vi "SSULE by Kamil Trajda.vi"() -> ()   [LabVIEW 2020]
uses:
  <vilib>/Utility/miscctls.llb/LVBoundsTypeDef.ctl
  <vilib>/Utility/inputDevices.llb/keyboardAcquire.vi
  <vilib>/Utility/inputDevices.llb/joystickAcquire.vi
  <vilib>/Utility/inputDevices.llb/closeJoystick.vi
  <vilib>/Utility/inputDevices.llb/closeKeyboard.vi
panel:
  out "?":bool
  in  "Przechodzenie przez ściany":bool
  in  "Rodzaj pada":string(combo)
  out "SCORE":i32
  in  "Prędkość węża":u32(slide)=150 min=150 max=200 step=1 scale=200.0..150.0
  in  "?":bool
  in  "Przechodzenie przez ściany":bool
  out "SUPER SNAKE ULTIMATE LABVIEW EDITION":picture
  # "SUPER SNAKE ULTIMATE LABVIEW EDITION !!!!"
  # "EXIT"
  # "OPCJE"
  # "Ściana"
  # "KONTROLA PADA"
  # "Używać pada?"
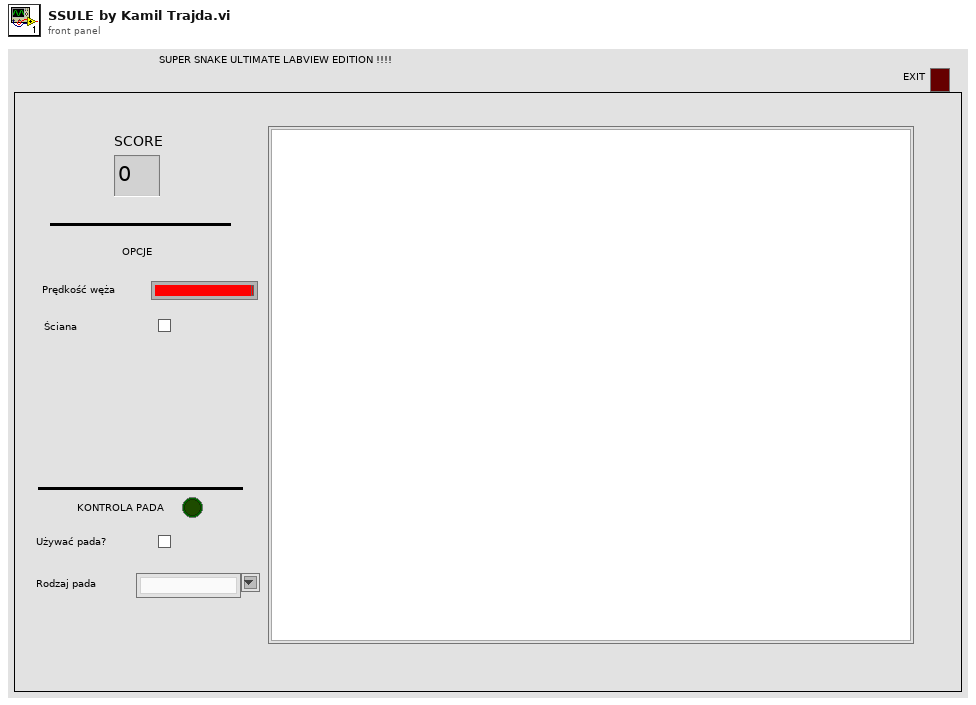
[diagram p1: front panel]
types:
  T1 = typedef "LVBoundsTypeDef.ctl" = cluster{"Width":u32, "Height":u32}
  T2 = cluster{"axes total":u32, "buttons total":u32, "pov total":u32, "device name":string}[]
  T3 = enum16{"0", "1", "2", "3", "4", "5", "6", "7", "8", "9", "A", "B", "C", "D", "E", "F", "G", "H", "I", "J", "K", "L", "M", "N", "O", "P", "Q", "R", "S", "T", "U", "V", "W", "X", "Y", "Z", "F1", "F2", "F3", "F4", "F5", "F6", "F7", "F8", "F9", "F10", "F11", "F12", "F13", "F14", "F15", "ADD", "BACK", "BACKSLASH", "CAPITAL", "COMMA", "DECIMAL", "DELETE", "DIVIDE", "DOWN", "END", "EQUALS", "ESCAPE", "GRAVE (`)", "HOME", "INSERT", "LBRACKET", "LCONTROL", "LEFT", "L ALT", "LSHIFT", "LWIN", "MINUS", "MULTIPLY", "NEXT", "NUMLOCK", "NUMPAD_0", "NUMPAD_1", "NUMPAD_2", "NUMPAD_3", "NUMPAD_4", "NUMPAD_5", "NUMPAD_6", "NUMPAD_7", "NUMPAD_8", "NUMPAD_9", "PAUSE", "PERIOD", "PRIOR (PG UP)", "RBRACKET", "RCONTROL", "RETURN", "RIGHT", "R ALT", "RSHIFT", "RWIN", "SCROLL", "SEMICOLON", "SLASH", "SPACE", "SUBTRACT", "TAB", "UP", "ENTER (num pad)", "' (quote)"}[]
  T4 = cluster{"keys pressed[0]":enum16{"0", "1", "2", "3", "4", "5", "6", "7", "8", "9", "A", "B", "C", "D", "E", "F", "G", "H", "I", "J", "K", "L", "M", "N", "O", "P", "Q", "R", "S", "T", "U", "V", "W", "X", "Y", "Z", "F1", "F2", "F3", "F4", "F5", "F6", "F7", "F8", "F9", "F10", "F11", "F12", "F13", "F14", "F15", "ADD", "BACK", "BACKSLASH", "CAPITAL", "COMMA", "DECIMAL", "DELETE", "DIVIDE", "DOWN", "END", "EQUALS", "ESCAPE", "GRAVE (`)", "HOME", "INSERT", "LBRACKET", "LCONTROL", "LEFT", "L ALT", "LSHIFT", "LWIN", "MINUS", "MULTIPLY", "NEXT", "NUMLOCK", "NUMPAD_0", "NUMPAD_1", "NUMPAD_2", "NUMPAD_3", "NUMPAD_4", "NUMPAD_5", "NUMPAD_6", "NUMPAD_7", "NUMPAD_8", "NUMPAD_9", "PAUSE", "PERIOD", "PRIOR (PG UP)", "RBRACKET", "RCONTROL", "RETURN", "RIGHT", "R ALT", "RSHIFT", "RWIN", "SCROLL", "SEMICOLON", "SLASH", "SPACE", "SUBTRACT", "TAB", "UP", "ENTER (num pad)", "' (quote)"}, "keys pressed[1]":enum16{"0", "1", "2", "3", "4", "5", "6", "7", "8", "9", "A", "B", "C", "D", "E", "F", "G", "H", "I", "J", "K", "L", "M", "N", "O", "P", "Q", "R", "S", "T", "U", "V", "W", "X", "Y", "Z", "F1", "F2", "F3", "F4", "F5", "F6", "F7", "F8", "F9", "F10", "F11", "F12", "F13", "F14", "F15", "ADD", "BACK", "BACKSLASH", "CAPITAL", "COMMA", "DECIMAL", "DELETE", "DIVIDE", "DOWN", "END", "EQUALS", "ESCAPE", "GRAVE (`)", "HOME", "INSERT", "LBRACKET", "LCONTROL", "LEFT", "L ALT", "LSHIFT", "LWIN", "MINUS", "MULTIPLY", "NEXT", "NUMLOCK", "NUMPAD_0", "NUMPAD_1", "NUMPAD_2", "NUMPAD_3", "NUMPAD_4", "NUMPAD_5", "NUMPAD_6", "NUMPAD_7", "NUMPAD_8", "NUMPAD_9", "PAUSE", "PERIOD", "PRIOR (PG UP)", "RBRACKET", "RCONTROL", "RETURN", "RIGHT", "R ALT", "RSHIFT", "RWIN", "SCROLL", "SEMICOLON", "SLASH", "SPACE", "SUBTRACT", "TAB", "UP", "ENTER (num pad)", "' (quote)"}, "keys pressed[2]":enum16{"0", "1", "2", "3", "4", "5", "6", "7", "8", "9", "A", "B", "C", "D", "E", "F", "G", "H", "I", "J", "K", "L", "M", "N", "O", "P", "Q", "R", "S", "T", "U", "V", "W", "X", "Y", "Z", "F1", "F2", "F3", "F4", "F5", "F6", "F7", "F8", "F9", "F10", "F11", "F12", "F13", "F14", "F15", "ADD", "BACK", "BACKSLASH", "CAPITAL", "COMMA", "DECIMAL", "DELETE", "DIVIDE", "DOWN", "END", "EQUALS", "ESCAPE", "GRAVE (`)", "HOME", "INSERT", "LBRACKET", "LCONTROL", "LEFT", "L ALT", "LSHIFT", "LWIN", "MINUS", "MULTIPLY", "NEXT", "NUMLOCK", "NUMPAD_0", "NUMPAD_1", "NUMPAD_2", "NUMPAD_3", "NUMPAD_4", "NUMPAD_5", "NUMPAD_6", "NUMPAD_7", "NUMPAD_8", "NUMPAD_9", "PAUSE", "PERIOD", "PRIOR (PG UP)", "RBRACKET", "RCONTROL", "RETURN", "RIGHT", "R ALT", "RSHIFT", "RWIN", "SCROLL", "SEMICOLON", "SLASH", "SPACE", "SUBTRACT", "TAB", "UP", "ENTER (num pad)", "' (quote)"}, "keys pressed[3]":enum16{"0", "1", "2", "3", "4", "5", "6", "7", "8", "9", "A", "B", "C", "D", "E", "F", "G", "H", "I", "J", "K", "L", "M", "N", "O", "P", "Q", "R", "S", "T", "U", "V", "W", "X", "Y", "Z", "F1", "F2", "F3", "F4", "F5", "F6", "F7", "F8", "F9", "F10", "F11", "F12", "F13", "F14", "F15", "ADD", "BACK", "BACKSLASH", "CAPITAL", "COMMA", "DECIMAL", "DELETE", "DIVIDE", "DOWN", "END", "EQUALS", "ESCAPE", "GRAVE (`)", "HOME", "INSERT", "LBRACKET", "LCONTROL", "LEFT", "L ALT", "LSHIFT", "LWIN", "MINUS", "MULTIPLY", "NEXT", "NUMLOCK", "NUMPAD_0", "NUMPAD_1", "NUMPAD_2", "NUMPAD_3", "NUMPAD_4", "NUMPAD_5", "NUMPAD_6", "NUMPAD_7", "NUMPAD_8", "NUMPAD_9", "PAUSE", "PERIOD", "PRIOR (PG UP)", "RBRACKET", "RCONTROL", "RETURN", "RIGHT", "R ALT", "RSHIFT", "RWIN", "SCROLL", "SEMICOLON", "SLASH", "SPACE", "SUBTRACT", "TAB", "UP", "ENTER (num pad)", "' (quote)"}, "keys pressed[4]":enum16{"0", "1", "2", "3", "4", "5", "6", "7", "8", "9", "A", "B", "C", "D", "E", "F", "G", "H", "I", "J", "K", "L", "M", "N", "O", "P", "Q", "R", "S", "T", "U", "V", "W", "X", "Y", "Z", "F1", "F2", "F3", "F4", "F5", "F6", "F7", "F8", "F9", "F10", "F11", "F12", "F13", "F14", "F15", "ADD", "BACK", "BACKSLASH", "CAPITAL", "COMMA", "DECIMAL", "DELETE", "DIVIDE", "DOWN", "END", "EQUALS", "ESCAPE", "GRAVE (`)", "HOME", "INSERT", "LBRACKET", "LCONTROL", "LEFT", "L ALT", "LSHIFT", "LWIN", "MINUS", "MULTIPLY", "NEXT", "NUMLOCK", "NUMPAD_0", "NUMPAD_1", "NUMPAD_2", "NUMPAD_3", "NUMPAD_4", "NUMPAD_5", "NUMPAD_6", "NUMPAD_7", "NUMPAD_8", "NUMPAD_9", "PAUSE", "PERIOD", "PRIOR (PG UP)", "RBRACKET", "RCONTROL", "RETURN", "RIGHT", "R ALT", "RSHIFT", "RWIN", "SCROLL", "SEMICOLON", "SLASH", "SPACE", "SUBTRACT", "TAB", "UP", "ENTER (num pad)", "' (quote)"}, "keys pressed[5]":enum16{"0", "1", "2", "3", "4", "5", "6", "7", "8", "9", "A", "B", "C", "D", "E", "F", "G", "H", "I", "J", "K", "L", "M", "N", "O", "P", "Q", "R", "S", "T", "U", "V", "W", "X", "Y", "Z", "F1", "F2", "F3", "F4", "F5", "F6", "F7", "F8", "F9", "F10", "F11", "F12", "F13", "F14", "F15", "ADD", "BACK", "BACKSLASH", "CAPITAL", "COMMA", "DECIMAL", "DELETE", "DIVIDE", "DOWN", "END", "EQUALS", "ESCAPE", "GRAVE (`)", "HOME", "INSERT", "LBRACKET", "LCONTROL", "LEFT", "L ALT", "LSHIFT", "LWIN", "MINUS", "MULTIPLY", "NEXT", "NUMLOCK", "NUMPAD_0", "NUMPAD_1", "NUMPAD_2", "NUMPAD_3", "NUMPAD_4", "NUMPAD_5", "NUMPAD_6", "NUMPAD_7", "NUMPAD_8", "NUMPAD_9", "PAUSE", "PERIOD", "PRIOR (PG UP)", "RBRACKET", "RCONTROL", "RETURN", "RIGHT", "R ALT", "RSHIFT", "RWIN", "SCROLL", "SEMICOLON", "SLASH", "SPACE", "SUBTRACT", "TAB", "UP", "ENTER (num pad)", "' (quote)"}, "keys pressed[6]":enum16{"0", "1", "2", "3", "4", "5", "6", "7", "8", "9", "A", "B", "C", "D", "E", "F", "G", "H", "I", "J", "K", "L", "M", "N", "O", "P", "Q", "R", "S", "T", "U", "V", "W", "X", "Y", "Z", "F1", "F2", "F3", "F4", "F5", "F6", "F7", "F8", "F9", "F10", "F11", "F12", "F13", "F14", "F15", "ADD", "BACK", "BACKSLASH", "CAPITAL", "COMMA", "DECIMAL", "DELETE", "DIVIDE", "DOWN", "END", "EQUALS", "ESCAPE", "GRAVE (`)", "HOME", "INSERT", "LBRACKET", "LCONTROL", "LEFT", "L ALT", "LSHIFT", "LWIN", "MINUS", "MULTIPLY", "NEXT", "NUMLOCK", "NUMPAD_0", "NUMPAD_1", "NUMPAD_2", "NUMPAD_3", "NUMPAD_4", "NUMPAD_5", "NUMPAD_6", "NUMPAD_7", "NUMPAD_8", "NUMPAD_9", "PAUSE", "PERIOD", "PRIOR (PG UP)", "RBRACKET", "RCONTROL", "RETURN", "RIGHT", "R ALT", "RSHIFT", "RWIN", "SCROLL", "SEMICOLON", "SLASH", "SPACE", "SUBTRACT", "TAB", "UP", "ENTER (num pad)", "' (quote)"}, "keys pressed[7]":enum16{"0", "1", "2", "3", "4", "5", "6", "7", "8", "9", "A", "B", "C", "D", "E", "F", "G", "H", "I", "J", "K", "L", "M", "N", "O", "P", "Q", "R", "S", "T", "U", "V", "W", "X", "Y", "Z", "F1", "F2", "F3", "F4", "F5", "F6", "F7", "F8", "F9", "F10", "F11", "F12", "F13", "F14", "F15", "ADD", "BACK", "BACKSLASH", "CAPITAL", "COMMA", "DECIMAL", "DELETE", "DIVIDE", "DOWN", "END", "EQUALS", "ESCAPE", "GRAVE (`)", "HOME", "INSERT", "LBRACKET", "LCONTROL", "LEFT", "L ALT", "LSHIFT", "LWIN", "MINUS", "MULTIPLY", "NEXT", "NUMLOCK", "NUMPAD_0", "NUMPAD_1", "NUMPAD_2", "NUMPAD_3", "NUMPAD_4", "NUMPAD_5", "NUMPAD_6", "NUMPAD_7", "NUMPAD_8", "NUMPAD_9", "PAUSE", "PERIOD", "PRIOR (PG UP)", "RBRACKET", "RCONTROL", "RETURN", "RIGHT", "R ALT", "RSHIFT", "RWIN", "SCROLL", "SEMICOLON", "SLASH", "SPACE", "SUBTRACT", "TAB", "UP", "ENTER (num pad)", "' (quote)"}, "keys pressed[8]":enum16{"0", "1", "2", "3", "4", "5", "6", "7", "8", "9", "A", "B", "C", "D", "E", "F", "G", "H", "I", "J", "K", "L", "M", "N", "O", "P", "Q", "R", "S", "T", "U", "V", "W", "X", "Y", "Z", "F1", "F2", "F3", "F4", "F5", "F6", "F7", "F8", "F9", "F10", "F11", "F12", "F13", "F14", "F15", "ADD", "BACK", "BACKSLASH", "CAPITAL", "COMMA", "DECIMAL", "DELETE", "DIVIDE", "DOWN", "END", "EQUALS", "ESCAPE", "GRAVE (`)", "HOME", "INSERT", "LBRACKET", "LCONTROL", "LEFT", "L ALT", "LSHIFT", "LWIN", "MINUS", "MULTIPLY", "NEXT", "NUMLOCK", "NUMPAD_0", "NUMPAD_1", "NUMPAD_2", "NUMPAD_3", "NUMPAD_4", "NUMPAD_5", "NUMPAD_6", "NUMPAD_7", "NUMPAD_8", "NUMPAD_9", "PAUSE", "PERIOD", "PRIOR (PG UP)", "RBRACKET", "RCONTROL", "RETURN", "RIGHT", "R ALT", "RSHIFT", "RWIN", "SCROLL", "SEMICOLON", "SLASH", "SPACE", "SUBTRACT", "TAB", "UP", "ENTER (num pad)", "' (quote)"}}
  T5 = enum16{"0", "1", "2", "3", "4", "5", "6", "7", "8", "9", "A", "B", "C", "D", "E", "F", "G", "H", "I", "J", "K", "L", "M", "N", "O", "P", "Q", "R", "S", "T", "U", "V", "W", "X", "Y", "Z", "F1", "F2", "F3", "F4", "F5", "F6", "F7", "F8", "F9", "F10", "F11", "F12", "F13", "F14", "F15", "ADD", "BACK", "BACKSLASH", "CAPITAL", "COMMA", "DECIMAL", "DELETE", "DIVIDE", "DOWN", "END", "EQUALS", "ESCAPE", "GRAVE (`)", "HOME", "INSERT", "LBRACKET", "LCONTROL", "LEFT", "L ALT", "LSHIFT", "LWIN", "MINUS", "MULTIPLY", "NEXT", "NUMLOCK", "NUMPAD_0", "NUMPAD_1", "NUMPAD_2", "NUMPAD_3", "NUMPAD_4", "NUMPAD_5", "NUMPAD_6", "NUMPAD_7", "NUMPAD_8", "NUMPAD_9", "PAUSE", "PERIOD", "PRIOR (PG UP)", "RBRACKET", "RCONTROL", "RETURN", "RIGHT", "R ALT", "RSHIFT", "RWIN", "SCROLL", "SEMICOLON", "SLASH", "SPACE", "SUBTRACT", "TAB", "UP", "ENTER (num pad)", "' (quote)"}
  T6 = cluster{"X axis":i32, "Y axis":i32, "Z axis":i32, "X axis rotation":i32, "Y axis rotation":i32, "Z axis rotation":i32, "U axis":i32, "V axis":i32}
  T7 = typedef "imagedata.ctl" = cluster{"image type":i32, "image depth":i32, "image":u8[], "mask":u8[], "colors":u32[], "Rectangle":cluster{"left":i16, "top":i16, "right":i16, "bottom":i16}}
  T8 = cluster{"image type":i32, "image depth":i32, "image":u8[], "mask":u8[], "colors":u32[], "Cluster":cluster{dbl, dbl, dbl, dbl}}
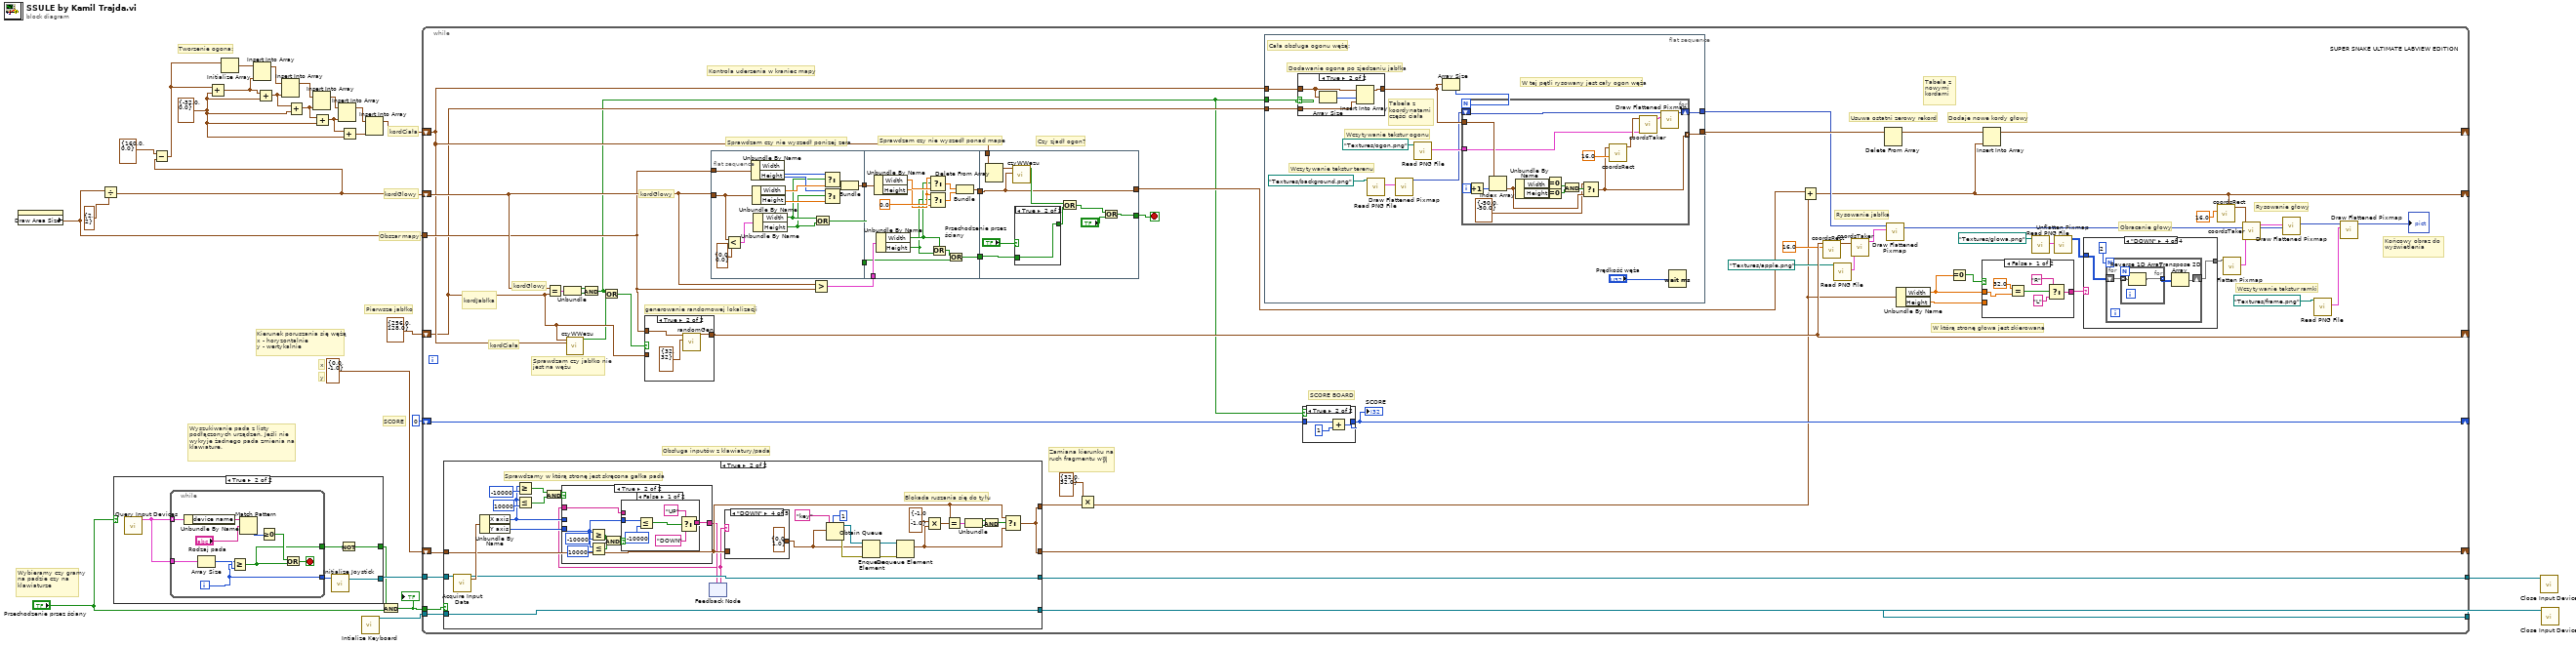
[diagram p0: block diagram]
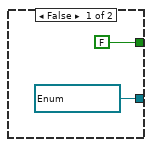
[diagram p2: hidden frame]
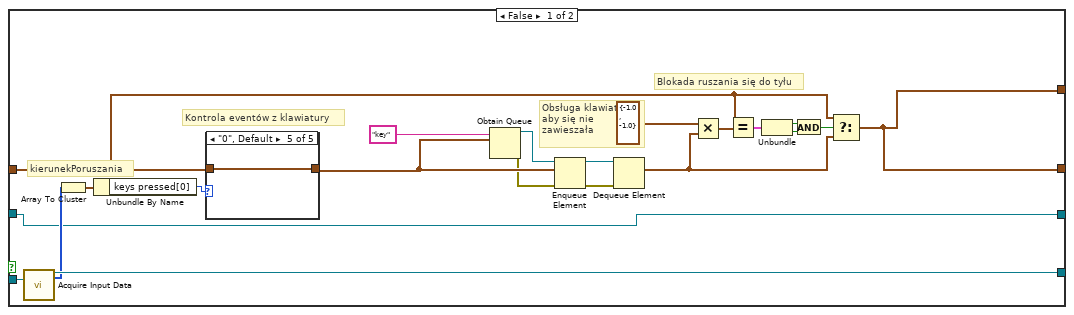
[diagram p3: hidden frame]
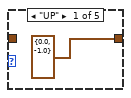
[diagram p4: hidden frame]
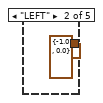
[diagram p5: hidden frame]
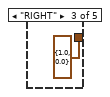
[diagram p6: hidden frame]
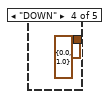
[diagram p7: hidden frame]
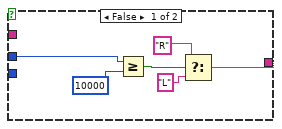
[diagram p8: hidden frame]
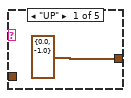
[diagram p10: hidden frame]
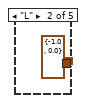
[diagram p11: hidden frame]
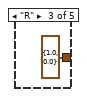
[diagram p12: hidden frame]
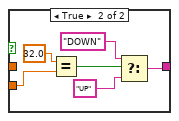
[diagram p15: hidden frame]
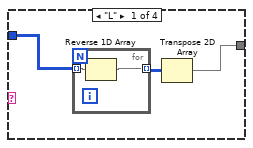
[diagram p16: hidden frame]
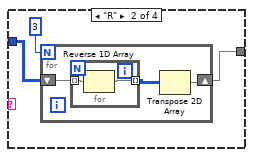
[diagram p17: hidden frame]
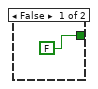
[diagram p20: hidden frame]
diagram:
  w16 = cluster{"Width":dbl, "Height":dbl} {"Width"=-32.0, "Height"=0.0} ("y")
  # "SCORE"
  # "Wyszukiwanie pada z listy podłączonych urządzeń. Jeśli nie wykryje żadnego pada zmienia na klawiature."
  # "Wybieramy czy gramy na padzie czy na klawiaturze"
  # "kordCiała"
  # "Obszar mapy"
  # "kordGlowy"
  # "Pierwsze jabłko"
  # "y"
  # "x"
  # "Kierunek poruszania się wężą\nx - horyzontalnie\ny - wertykalnie"
  # "Tworzenie ogona:"
  n1 = property class="Pict"() -> ("Draw Area Size"=w26:T1)  [unwired: 2 in, 2 out]
  n2 = Divide(x=w26, y=T1 {"Width"=2, "Height"=2}) -> (x/y=w10:cluster{"Width":dbl, "Height":dbl})
  n3 = case shown="True" "Przechodzenie przez ściany" {
    tunnel: [w29 w34] -> w6
    tunnel: [FALSE w31] -> w3
    frame False {
      w29 = refnum<k1> refnum items=["JOYSTICK"] ("device ID")
    }
    frame True {
      n4 = call <vilib>:"Query Input Devices.vi"() -> ("joystick info"=w33:T2)  [unwired: 8 in, 3 out]
      n5 = while {
        tunnel: w33 -> [w42] mode=indexing
        tunnel: w33 -> [w44]
        tunnel: [w38] -> w30
        tunnel: [w36] -> w32
        i -> [w36]
        stop <- w40 stop-if-true
        n6 = Unbundle By Name(w42) -> ("device name"=w35:string)
        n7 = Array Size(array=w44) -> (size(s)=w37:i32)
        n8 = Greater Or Equal?(x=w36, y=w37) -> (x >= y?=w38:bool)
        n9 = Match Pattern(string=w35, regular expression="Rodzaj pada") -> (offset past match=w41:i32)  [unwired: 1 in, 3 out]
        n10 = Greater Or Equal To 0?(x=w41) -> (x >= 0?=w39:bool)
        n11 = Or(x=w39, y=w38) -> (x .or. y?=w40:bool)
      }
      n12 = call <vilib>:"Initialize Joystick.vi"("device index"=w32) -> ("device ID"=w34:refnum<k1>)  [unwired: 9 in, 1 out]
      n13 = Not(x=w30) -> (.not. x?=w31:bool)
    }
  }
  n14 = Subtract(x=cluster{"Width":dbl, "Height":dbl} {"Width"=160.0, "Height"=0.0} ("y"), y=w10) -> (x-y=w8:cluster{"Width":dbl, "Height":dbl})
  n15 = Add(x=w8, y=w16) -> (x+y=w21:cluster{"Width":dbl, "Height":dbl})
  n16 = Initialize Array(w8) -> (w23:cluster{"Width":dbl, "Height":dbl}[])  [unwired: 1 in]
  n17 = Insert Into Array(array=w23, new element=w21) -> (w22:cluster{"Width":dbl, "Height":dbl}[])  [unwired: 1 in]
  n18 = Add(x=w21, y=w16) -> (x+y=w19:cluster{"Width":dbl, "Height":dbl})
  n19 = Insert Into Array(array=w22, new element=w19) -> (w15:cluster{"Width":dbl, "Height":dbl}[])  [unwired: 1 in]
  n20 = Add(x=w19, y=w16) -> (x+y=w18:cluster{"Width":dbl, "Height":dbl})
  n21 = Insert Into Array(array=w15, new element=w18) -> (w14:cluster{"Width":dbl, "Height":dbl}[])  [unwired: 1 in]
  n22 = Add(x=w18, y=w16) -> (x+y=w17:cluster{"Width":dbl, "Height":dbl})
  n23 = Insert Into Array(array=w14, new element=w17) -> (w13:cluster{"Width":dbl, "Height":dbl}[])  [unwired: 1 in]
  n24 = Add(x=w17, y=w16) -> (x+y=w20:cluster{"Width":dbl, "Height":dbl})
  n25 = call <vilib>:"Intialize Keyboard.vi"() -> ("device ID"=w4:refnum<k1>)  [unwired: 10 in, 1 out]
  n26 = Insert Into Array(array=w13, new element=w20) -> (w12:cluster{"Width":dbl, "Height":dbl}[])  [unwired: 1 in]
  n27 = And(x=w3, y="Przechodzenie przez ściany") -> (x .and. y?=w1:bool)
  "?" <- w1
  n28 = while {
    shift-right: [w60] -> _
    shift-left: w10 -> [w95]
    tunnel: w26 -> [w94]
    tunnel: w4 -> [w101]
    tunnel: [w100] -> w25
    shift-right: [w96] -> _
    shift-left: cluster{"Width":dbl, "Height":dbl} {"Width"=0.0, "Height"=-1.0} ("y") -> [w97]
    shift-right: [w99] -> _
    shift-left: w12 -> [w93]
    shift-right: [w67] -> _
    shift-left: cluster{dbl, dbl} {256.0, 128.0} -> [w92]
    shift-right: [w55] -> _
    shift-left: 0 -> [w56]
    tunnel: w6 -> [w50]
    tunnel: w1 -> [w49]
    tunnel: [w48] -> w5
    stop <- w79 stop-if-true
    # "Końcowy obraz do wyświetlenia"
    # "Zamiana kierunku na ruch fragmentu w꿹"
    # "Obsługa inputów z klawiatury/pada"
    # "Wczytywanie tekstur ramki"
    # "SCORE BOARD"
    # "Obracanie głowy"
    # "W którą stronę głowa jest skierowana"
    # "Rysowanie jabłka"
    # "Czy zjadł ogon?"
    # "Sprawdzam czy nie wyszedł ponizej zera"
    # "Sprawdzam czy nie wyszedł ponad mape"
    # "kordCiała"
    # "kordJabłka"
    # "kordGlowy"
    # "kordGlowy"
    # "Sprawdzam czy jabłko nie jest na wężu"
    # "generowanie randomowej lokalizacji"
    # "Kontrola uderzenia w kraniec mapy"
    # "Dodaje nowe kordy głowy"
    # "Usuwa ostatni zerowy rekord"
    # "Tabela z nowymi kordami"
    # "Rysowanie głowy"
    n29 = case shown="True" w49 {
      tunnel: w101 -> [w122 w154]
      tunnel: [w121 w154] -> w100
      tunnel: w97 -> [w105 w138]
      tunnel: [w102 w139] -> w96
      tunnel: [w102 w139] -> w46
      tunnel: w50 -> [w103 w156]
      tunnel: [w103 w153] -> w48
      frame False {
        # "kierunekPoruszania"
        # "Blokada ruszania się do tyłu"
        # "Obsługa klawiatury, aby się nie zawieszała"
        # "Kontrola eventów z klawiatury"
        n30 = call-poly <vilib>:"Acquire Input Data.vi"("device ID"=w122) -> ("device ID"=w121:refnum<k1>, "keys pressed"=w120:T3)  [unwired: 16 in, 1 out]
        n31 = Array To Cluster(array=w120) -> (cluster=w119:T4)
        n32 = Unbundle By Name(w119) -> ("keys pressed[0]"=w118:T5)
        n33 = case shown="\"0\", Default" w118 {
          tunnel: [cluster{"Width":dbl, "Height":dbl} {"Width"=0.0, "Height"=-1.0} ("y") cluster{"Width":dbl, "Height":dbl} {"Width"=-1.0, "Height"=0.0} ("y") cluster{"Width":dbl, "Height":dbl} {"Width"=1.0, "Height"=0.0} ("y") cluster{"Width":dbl, "Height":dbl} {"Width"=0.0, "Height"=1.0} ("y") w127] -> w117
          tunnel: w105 -> [_ _ _ _ w127]
          frame "UP" {
          }
          frame "LEFT" {
          }
          frame "RIGHT" {
          }
          frame "DOWN" {
          }
          frame "0", Default {
          }
        }
        n34 = Obtain Queue(name (unnamed)="key", element data type=w117) -> (queue out=w116:refnum<queue>, error out=w114:errorcluster)  [unwired: 3 in, 1 out]
        n35 = Enqueue Element(queue=w116, element=w117, error in (no error)=w114) -> (queue out=w115:refnum<queue>, error out=w113:errorcluster)  [unwired: 1 in, 1 out]
        n36 = Dequeue Element(queue=w115, error in (no error)=w113) -> (element=w104:cluster{"Width":dbl, "Height":dbl})  [unwired: 1 in, 3 out]
        n37 = Multiply(x=cluster{"Width":dbl, "Height":dbl} {"Width"=-1.0, "Height"=-1.0}, y=w104) -> (x*y=w111:cluster{"Width":dbl, "Height":dbl})
        n38 = Equal?(x=w105, y=w111) -> (x = y?=w107:cluster{"Width":bool, "Height":bool})
        n39 = Unbundle(w107) -> ("Width"=w109:bool, "Height"=w108:bool)
        n40 = And(x=w109, y=w108) -> (x .and. y?=w106:bool)
        n41 = Select(t=w105, s=w106, f=w104) -> (s? t:f=w102:cluster{"Width":dbl, "Height":dbl})
      }
      frame True {
        # "Sprawdzamy w którą stronę jest skręcona gałka pada"
        # "Blokada ruszania się do tyłu"
        n42 = call-poly <vilib>:"Acquire Input Data.vi"("device ID"=w156) -> ("device ID"=w153:refnum<k1>, "axis info"=w155:T6)  [unwired: 14 in, 3 out]
        n43 = Unbundle By Name(w155) -> ("X axis"=w147:i32, "Y axis"=w146:i32)
        n44 = Greater Or Equal?(x=w147, y=-10000) -> (x >= y?=w152:bool)
        n45 = Less Or Equal?(x=w147, y=10000) -> (x <= y?=w151:bool)
        n46 = And(x=w152, y=w151) -> (x .and. y?=w148:bool)
        n47 = feedback #1() -> (w129:string)  [unwired: 1 in]
        n48 = case shown="True" w148 {
          tunnel: w147 -> [w157 _]
          tunnel: w146 -> [_ w165]
          tunnel: [w160 w164] -> w130
          tunnel: w129 -> [_ w163]
          frame False {
            n49 = Greater Or Equal?(x=w157, y=10000) -> (x >= y?=w158:bool)
            n50 = Select(t="R", s=w158, f="L") -> (s? t:f=w160:string)
          }
          frame True {
            n51 = Greater Or Equal?(x=w165, y=-10000) -> (x >= y?=w170:bool)
            n52 = Less Or Equal?(x=w165, y=10000) -> (x <= y?=w169:bool)
            n53 = And(x=w170, y=w169) -> (x .and. y?=w166:bool)
            n54 = case shown="False" w166 {
              tunnel: w165 -> [w172 _]
              tunnel: [w171 w177] -> w164
              tunnel: w163 -> [_ w177]
              frame False {
                n55 = Less Or Equal?(x=w172, y=-10000) -> (x <= y?=w176:bool)
                n56 = Select(t="UP", s=w176, f="DOWN") -> (s? t:f=w171:string)
              }
              frame True {
              }
            }
          }
        }
        n57 = feedback-in #1(w130) -> ()
        n58 = case shown="\"DOWN\"" w129 {
          tunnel: [cluster{"Width":dbl, "Height":dbl} {"Width"=0.0, "Height"=-1.0} ("y") cluster{"Width":dbl, "Height":dbl} {"Width"=-1.0, "Height"=0.0} ("y") cluster{"Width":dbl, "Height":dbl} {"Width"=1.0, "Height"=0.0} ("y") cluster{"Width":dbl, "Height":dbl} {"Width"=0.0, "Height"=1.0} ("y") w182] -> w132
          tunnel: w138 -> [_ _ _ _ w182]
          frame "UP" {
          }
          frame "L" {
          }
          frame "R" {
          }
          frame "DOWN" {
          }
          frame "0", Default {
          }
        }
        n59 = Obtain Queue(max queue size (-1, unlimited)=1, name (unnamed)="key", element data type=w132) -> (queue out=w137:refnum<queue>, error out=w135:errorcluster)  [unwired: 2 in, 1 out]
        n60 = Enqueue Element(queue=w137, element=w132, error in (no error)=w135) -> (queue out=w136:refnum<queue>, error out=w134:errorcluster)  [unwired: 1 in, 1 out]
        n61 = Dequeue Element(queue=w136, error in (no error)=w134) -> (element=w131:cluster{"Width":dbl, "Height":dbl})  [unwired: 1 in, 3 out]
        n62 = Multiply(x=cluster{"Width":dbl, "Height":dbl} {"Width"=-1.0, "Height"=-1.0}, y=w131) -> (x*y=w145:cluster{"Width":dbl, "Height":dbl})
        n63 = Equal?(x=w138, y=w145) -> (x = y?=w141:cluster{"Width":bool, "Height":bool})
        n64 = Unbundle(w141) -> ("Width"=w143:bool, "Height"=w142:bool)
        n65 = And(x=w143, y=w142) -> (x .and. y?=w140:bool)
        n66 = Select(t=w138, s=w140, f=w131) -> (s? t:f=w139:cluster{"Width":dbl, "Height":dbl})
      }
    }
    n67 = Equal?(x=w95, y=w92) -> (x = y?=w85:cluster{bool, bool})
    n68 = Unbundle(w85) -> (w84:bool, w83:bool)
    n69 = call "czyWWezu.vi"("kordyPunktu"=w92, "kordyCiala"=w93) -> ("czyNaszedl?"=w81:bool)  [unwired: 9 in]
    n70 = And(x=w84, y=w83) -> (x .and. y?=w57:bool)
    n71 = Or(x=w57, y=w81) -> (x .or. y?=w82:bool)
    n72 = case shown="True" w82 {
      tunnel: w94 -> [_ w298]
      tunnel: [w295 w297] -> w67
      tunnel: w92 -> [w295 _]
      frame False {
      }
      frame True {
        n73 = call "randomGen.vi"("dzielnikMapy"=T1 {"Width"=32, "Height"=32} ("y"), "Wielkosc mapy"=w298) -> ("wygenerowane współrzędne"=w297:cluster{u64, u64})  [unwired: 9 in]
      }
    }
    n74 = flat-sequence {
      tunnel: w94 -> [w269]
      tunnel: w95 -> [w259]
      tunnel: [w262] -> w89
      tunnel: [w256] -> w88
      tunnel: w89 -> [w278]
      tunnel: w80 -> [w282]
      tunnel: [w279] -> w87
      tunnel: w88 -> [w271]
      tunnel: [w270] -> w86
      tunnel: [w289] -> w90
      tunnel: w87 -> [w289]
      tunnel: w93 -> [w291]
      tunnel: w86 -> [w287]
      tunnel: [w283] -> w79
      frame #0 {
        n75 = Less?(x=w259, y=cluster{"Width":dbl, "Height":dbl} {"Width"=0.0, "Height"=0.0}) -> (x < y?=w261:cluster{"Width":bool, "Height":bool})
        n76 = Unbundle By Name(w269) -> ("Width"=w268:u32, "Height"=w265:u32)
        n77 = Unbundle By Name(w259) -> ("Width"=w267:dbl, "Height"=w266:dbl)
        n78 = Unbundle By Name(w261) -> ("Width"=w258:bool, "Height"=w257:bool)
        n79 = Or(x=w258, y=w257) -> (x .or. y?=w256:bool)
        n80 = Select(t=w268, s=w258, f=w267) -> (s? t:f=w264:dbl)
        n81 = Select(t=w265, s=w257, f=w266) -> (s? t:f=w263:dbl)
        n82 = Bundle("Width"=w264, "Height"=w263) -> (w262:cluster{"Width":dbl, "Height":dbl})  [unwired: 1 in]
      }
      frame #1 {
        w276 = 0.0 ("f")
        n83 = Unbundle By Name(w278) -> ("Width"=w277:dbl, "Height"=w275:dbl)
        n84 = Unbundle By Name(w282) -> ("Width"=w274:bool, "Height"=w273:bool)
        n85 = Select(t=w276, s=w274, f=w277) -> (s? t:f=w281:dbl)
        n86 = Select(t=w276, s=w273, f=w275) -> (s? t:f=w280:dbl)
        n87 = Or(x=w274, y=w273) -> (x .or. y?=w272:bool)
        n88 = Or(x=w272, y=w271) -> (x .or. y?=w270:bool)
        n89 = Bundle("Width"=w281, "Height"=w280) -> (w279:cluster{"Width":dbl, "Height":dbl})  [unwired: 1 in]
      }
      frame #2 {
        n90 = Delete From Array(array=w291) -> (array with subset deleted=w292:cluster{"Width":dbl, "Height":dbl}[])  [unwired: 2 in, 1 out]
        n91 = call "czyWWezu.vi"("kordyPunktu"=w289, "kordyCiala"=w292) -> ("czyNaszedl?"=w290:bool)  [unwired: 9 in]
        n92 = case shown="True" "Przechodzenie przez ściany" {
          tunnel: w287 -> [_ w294]
          tunnel: [FALSE w294] -> w286
          frame False {
          }
          frame True {
          }
        }
        n93 = Or(x=w290, y=w286) -> (x .or. y?=w284:bool)
        n94 = Or(x=w284, y="?") -> (x .or. y?=w283:bool)
      }
    }
    n95 = Greater?(x=w95, y=w94) -> (0:w80:cluster{"Width":bool, "Height":bool})
    n96 = Multiply(x=cluster{"Width":dbl, "Height":dbl} {"Width"=32.0, "Height"=32.0} ("y"), y=w46) -> (x*y=w45:cluster{"Width":dbl, "Height":dbl})
    n97 = flat-sequence {
      tunnel: w57 -> [w233]
      tunnel: w93 -> [w232]
      tunnel: w92 -> [w231]
      tunnel: [w230] -> w62
      tunnel: [w229] -> w91
      frame #0 {
        # "Wczytywanie tekstur ogonu"
        # "Wczytywanie tekstur terenu"
        # "Dodawanie ogona po zjedzeniu jabłka"
        # "Tabela z koordynatami\nczęści ciała"
        # "W tej pętli rysowany jest cały ogon węża"
        # "Cała obsługa ogonu wężą:"
        n98 = case shown="True" w233 {
          tunnel: w232 -> [w234 w236]
          tunnel: [w234 w238] -> w228
          tunnel: w231 -> [_ w235]
          frame False {
          }
          frame True {
            n99 = Array Size(array=w236) -> (size(s)=w237:i32)
            n100 = Insert Into Array(array=w236, index=w237, new element=w235) -> (w238:cluster{"Width":dbl, "Height":dbl}[])
          }
        }
        n101 = call <vilib>:"Read PNG File.vi"("path to PNG file"=path "Textures/background.png") -> ("image data"=w223:T7)  [unwired: 8 in, 2 out]
        n102 = call <vilib>:"Draw Flattened Pixmap.vi"("image data"=w223) -> ("new picture"=w221:picture)  [unwired: 8 in]
        n103 = call <vilib>:"Read PNG File.vi"("path to PNG file"=path "Textures/ogon.png") -> ("image data"=w224:T7)  [unwired: 8 in, 2 out]
        n104 = Array Size(array=w228) -> (size(s)=w227:i32)
        n105 = for {
          N: w227 -> [_]
          shift-right: [w240] -> w230
          shift-left: w221 -> [w241]
          tunnel: w228 -> [w255]
          tunnel: [w244] -> w229 mode=indexing
          tunnel: w224 -> [w239]
          i -> [w253]
          n106 = Increment(x=w253) -> (x+1=w254:i32)
          n107 = Index Array(array=w255, index=w254) -> (element=w247:cluster{"Width":dbl, "Height":dbl})
          n108 = Unbundle By Name(w247) -> ("Width"=w252:dbl, "Height"=w251:dbl)
          n109 = Equal To 0?(x=w252) -> (x = 0?=w250:bool)
          n110 = Equal To 0?(x=w251) -> (x = 0?=w249:bool)
          n111 = And(x=w250, y=w249) -> (x .and. y?=w248:bool)
          n112 = Select(t=cluster{"Width":dbl, "Height":dbl} {"Width"=-50.0, "Height"=-50.0}, s=w248, f=w247) -> (s? t:f=w244:cluster{"Width":dbl, "Height":dbl})
          n113 = call "coordsRect.vi"("Rozmiar"=16.0 ("liczba"), "coords"=w244) -> ("Cluster"=w242:cluster{dbl, dbl, dbl, dbl})  [unwired: 9 in]
          n114 = call "coordsTaker.vi"("image data"=w239, "coords"=w242) -> ("Cluster out"=w243:T8)  [unwired: 9 in]
          n115 = call <vilib>:"Draw Flattened Pixmap.vi"("image data"=w243, "picture"=w241) -> ("new picture"=w240:picture)  [unwired: 7 in]
        }
        n116 = Wait (ms)(milliseconds to wait="Prędkość węża") -> ()  [unwired: 1 out]
      }
    }
    n117 = case shown="True" w57 {
      tunnel: w56 -> [w183 w186]
      tunnel: [w183 w185] -> w55
      frame False {
      }
      frame True {
        n118 = Add(x=w186, y=1) -> (x+y=w185:i32)
      }
    }
    "SCORE" <- w55
    n119 = Add(x=w90, y=w45) -> (x+y=w60:cluster{"Width":dbl, "Height":dbl})
    n120 = call "coordsRect.vi"("Rozmiar"=16.0, "coords"=w67) -> ("Cluster"=w64:cluster{dbl, dbl, dbl, dbl})  [unwired: 9 in]
    n121 = call <vilib>:"Read PNG File.vi"("path to PNG file"=path "Textures/apple.png") -> ("image data"=w59:T7)  [unwired: 8 in, 2 out]
    n122 = call "coordsTaker.vi"("image data"=w59, "coords"=w64) -> ("Cluster out"=w61:T8)  [unwired: 9 in]
    n123 = Delete From Array(array=w91) -> (array with subset deleted=w98:cluster{"Width":dbl, "Height":dbl}[])  [unwired: 2 in, 1 out]
    n124 = call <vilib>:"Draw Flattened Pixmap.vi"("image data"=w61, "picture"=w62) -> ("new picture"=w63:picture)  [unwired: 7 in]
    n125 = Unbundle By Name(w45) -> ("Width"=w69:dbl, "Height"=w70:dbl)
    n126 = Equal To 0?(x=w69) -> (x = 0?=w71:bool)
    n127 = case shown="False" w71 {
      tunnel: w70 -> [_ w197]
      tunnel: [w189 w193] -> w68
      tunnel: w69 -> [w190 _]
      frame False {
        n128 = Equal?(x=32.0, y=w190) -> (x = y?=w192:bool)
        n129 = Select(t="R", s=w192, f="L") -> (s? t:f=w189:string)
      }
      frame True {
        n130 = Equal?(x=32.0, y=w197) -> (x = y?=w198:bool)
        n131 = Select(t="DOWN", s=w198, f="UP") -> (s? t:f=w193:string)
      }
    }
    n132 = Insert Into Array(array=w98, new element=w60) -> (w99:cluster{"Width":dbl, "Height":dbl}[])  [unwired: 1 in]
    n133 = call <vilib>:"Read PNG File.vi"("path to PNG file"=path "Textures/glowa.png") -> ("image data"=w73:T7)  [unwired: 8 in, 2 out]
    n134 = call <vilib>:"Unflatten Pixmap.vi"("image data"=w73) -> ("24-bit pixmap"=w75:u32[][])  [unwired: 4 in, 6 out]
    n135 = case shown="\"DOWN\"" w68 {
      tunnel: w75 -> [w201 w205 w212 w214]
      tunnel: [w199 w204 w212 w213] -> w74
      frame "L" {
        n136 = for {
          tunnel: w201 -> [w203] mode=indexing
          tunnel: [w202] -> w200 mode=indexing
          n137 = Reverse 1D Array(array=w203) -> (reversed array=w202:u32[])
        }
        n138 = Transpose 2D Array(2D array=w200) -> (transposed array=w199:u32[][])
      }
      frame "R" {
        n139 = for {
          N: 3 -> [_]
          shift-right: [w207] -> w204
          shift-left: w205 -> [w209]
          n140 = for {
            tunnel: w209 -> [w211] mode=indexing
            tunnel: [w210] -> w208 mode=indexing
            n141 = Reverse 1D Array(array=w211) -> (reversed array=w210:u32[])
          }
          n142 = Transpose 2D Array(2D array=w208) -> (transposed array=w207:u32[][])
        }
      }
      frame "UP", Default {
      }
      frame "DOWN" {
        n143 = for {
          N: 2 -> [_]
          shift-right: [w216] -> w213
          shift-left: w214 -> [w218]
          n144 = for {
            tunnel: w218 -> [w220] mode=indexing
            tunnel: [w219] -> w217 mode=indexing
            n145 = Reverse 1D Array(array=w220) -> (reversed array=w219:u32[])
          }
          n146 = Transpose 2D Array(2D array=w217) -> (transposed array=w216:u32[][])
        }
      }
    }
    n147 = call "coordsRect.vi"("Rozmiar"=16.0 ("liczba"), "coords"=w60) -> ("Cluster"=w77:cluster{dbl, dbl, dbl, dbl})  [unwired: 9 in]
    n148 = call <vilib>:"Flatten Pixmap.vi"("24-bit pixmap"=w74) -> ("image data"=w58:T7)  [unwired: 10 in]
    n149 = call "coordsTaker.vi"("image data"=w58, "coords"=w77) -> ("Cluster out"=w72:T8)  [unwired: 9 in]
    n150 = call <vilib>:"Draw Flattened Pixmap.vi"("image data"=w72, "picture"=w63) -> ("new picture"=w52:picture)  [unwired: 7 in]
    n151 = call <vilib>:"Read PNG File.vi"("path to PNG file"=path "Textures/frame.png") -> ("image data"=w54:T7)  [unwired: 8 in, 2 out]
    n152 = call <vilib>:"Draw Flattened Pixmap.vi"("image data"=w54, "picture"=w52) -> ("new picture"=→"SUPER SNAKE ULTIMATE LABVIEW EDITION":picture)  [unwired: 7 in]
  }
  n153 = call-poly <vilib>:"Close Input Device.vi"("device ID"=w5) -> ()  [unwired: 9 in, 1 out]
  n154 = call-poly <vilib>:"Close Input Device.vi"("device ID"=w25) -> ()  [unwired: 9 in, 1 out]
